vi "valves_openinlets.vi"(4 "error in":errorcluster, 7 "COM4 in":refnum<k24>) -> (0 "error out":errorcluster, 3 "COM4 out":refnum<k24>)   [LabVIEW 2018]
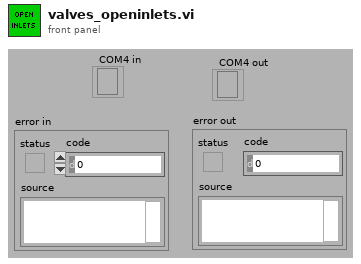
[diagram p1: front panel]
types:
  T1 = cluster{"Op A":u8[], "Op B":u8[], "Op C":u8[], "open":u8[], "L 3 A":u8[], "L 4 A 16":u8[], "F1 A":u8[], "L 4 A 34":u8[], "L 4 A 5":u8[], "FPw1 A":u8[], "L 2 A":u8[], "L 1 C FS":u8[], "L 2 C FS":u8[], "L 4 C 456 FS":u8[], "L 4 C 123 FS":u8[], "L 1 A":u8[], "L 1 C":u8[], "L 2 C":u8[], "L 4 C 456":u8[], "L 4 C 123":u8[], "FPw1 C":u8[], "F1 B":u8[], "F1 C":u8[], "F2 C":u8[], "F5 C":u8[]}
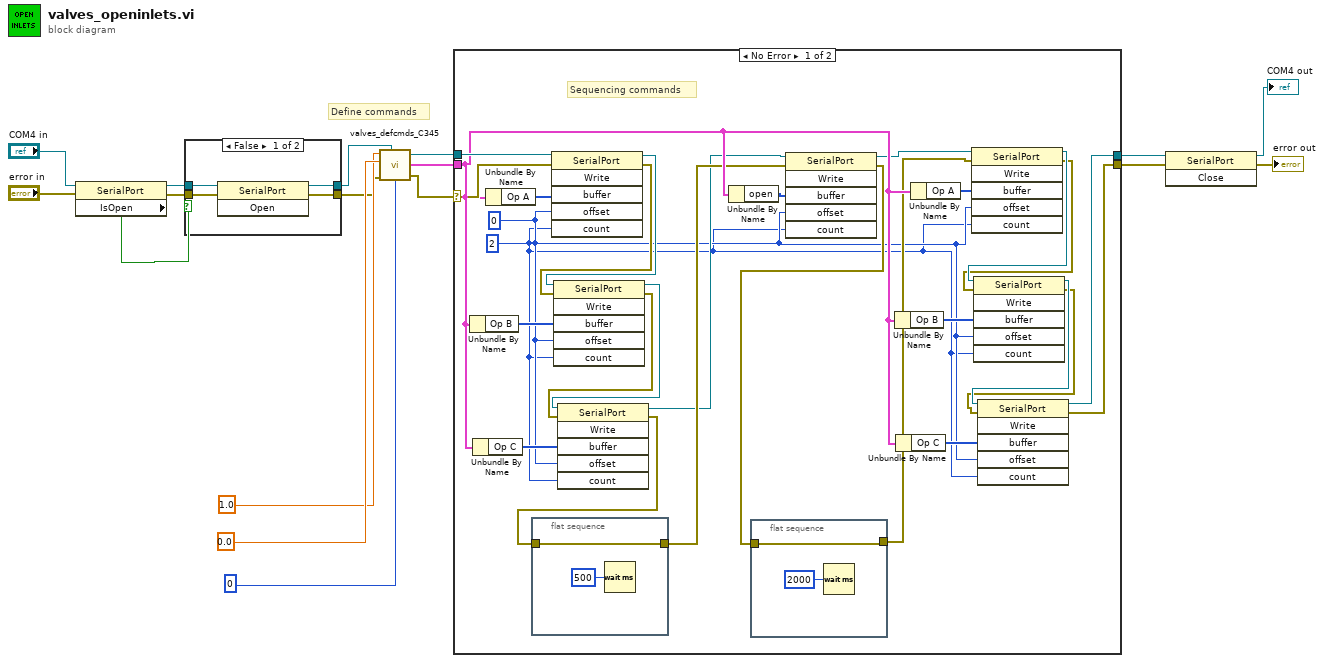
[diagram p0: block diagram]
diagram:
  # "Define commands"
  n1 = property class="SerialPort"(reference="COM4 in", error in="error in") -> (reference out=w5:refnum<k24>, error out=w6:errorcluster, "IsOpen"=w7:bool)
  n2 = case shown="False" w7 {
    tunnel: [w18 w23] -> w2
    tunnel: [w19 w22] -> w1
    tunnel: w6 -> [w20 w22]
    tunnel: w5 -> [w21 w23]
    frame False {
      n3 = invoke class="SerialPort" method="Open"(reference=w21, error in=w20) -> (reference out=w18:refnum<k24>, error out=w19:errorcluster)  [unwired: 1 in, 1 out]
    }
    frame True {
    }
  }
  n4 = call "valves_defcmds_C345.vi"("Input solution"=1.0, "Add to C"=0.0, "Rings to open"=u32 0, "error in"=w1, "COM4 in"=w2) -> ("COM4 out"=w13:refnum<k24>, "Commands out"=w16:T1, "error out"=w17:errorcluster)
  n5 = case shown="No Error" w17 {
    selector: w17 -> [w46 w57]
    tunnel: w13 -> [w51 w56]
    tunnel: [w33 w57] -> w14
    tunnel: w16 -> [w45 _]
    tunnel: [w38 w56] -> w12
    frame No Error {
      w24 = 2 ("count")
      w25 = 0 ("offset")
      # "Sequencing commands"
      n6 = Unbundle By Name(w45) -> ("Op B"=w31:u8[])
      n7 = Unbundle By Name(w45) -> ("Op C"=w32:u8[])
      n8 = Unbundle By Name(w45) -> ("Op A"=w30:u8[])
      n9 = flat-sequence {
        tunnel: [w54] -> w43
        tunnel: w44 -> [w54]
        frame #0 {
          n10 = Wait (ms)(milliseconds to wait=u32 500) -> ()  [unwired: 1 out]
        }
      }
      n11 = invoke class="SerialPort" method="Write"(reference=w51, error in=w46, "buffer"=w30, "offset"=w25, "count"=w24) -> (reference out=w50:refnum<k24>, error out=w49:errorcluster)  [unwired: 1 in, 4 out]
      n12 = invoke class="SerialPort" method="Write"(reference=w50, error in=w49, "buffer"=w31, "offset"=w25, "count"=w24) -> (reference out=w48:refnum<k24>, error out=w47:errorcluster)  [unwired: 1 in, 4 out]
      n13 = invoke class="SerialPort" method="Write"(reference=w48, error in=w47, "buffer"=w32, "offset"=w25, "count"=w24) -> (reference out=w42:refnum<k24>, error out=w44:errorcluster)  [unwired: 1 in, 4 out]
      n14 = Unbundle By Name(w45) -> ("open"=w29:u8[])
      n15 = flat-sequence {
        tunnel: [w52] -> w36
        tunnel: w37 -> [w52]
        frame #0 {
          n16 = Wait (ms)(milliseconds to wait=u32 2000) -> ()  [unwired: 1 out]
        }
      }
      n17 = invoke class="SerialPort" method="Write"(reference=w42, error in=w43, "buffer"=w29, "offset"=w25, "count"=w24) -> (reference out=w41:refnum<k24>, error out=w37:errorcluster)  [unwired: 1 in, 4 out]
      n18 = Unbundle By Name(w45) -> ("Op B"=w27:u8[])
      n19 = Unbundle By Name(w45) -> ("Op C"=w26:u8[])
      n20 = Unbundle By Name(w45) -> ("Op A"=w28:u8[])
      n21 = invoke class="SerialPort" method="Write"(reference=w41, error in=w36, "buffer"=w28, "offset"=w25, "count"=w24) -> (reference out=w40:refnum<k24>, error out=w35:errorcluster)  [unwired: 1 in, 4 out]
      n22 = invoke class="SerialPort" method="Write"(reference=w40, error in=w35, "buffer"=w27, "offset"=w25, "count"=w24) -> (reference out=w39:refnum<k24>, error out=w34:errorcluster)  [unwired: 1 in, 4 out]
      n23 = invoke class="SerialPort" method="Write"(reference=w39, error in=w34, "buffer"=w26, "offset"=w25, "count"=w24) -> (reference out=w38:refnum<k24>, error out=w33:errorcluster)  [unwired: 1 in, 4 out]
    }
    frame Error {
    }
  }
  n24 = invoke class="SerialPort" method="Close"(reference=w12, error in=w14) -> (reference out=→"COM4 out":refnum<k24>, error out=→"error out":errorcluster)  [unwired: 1 in, 1 out]
